vi "ROI entry-Offset ROI (core).vi"(9 "Function":T1=enum."Offset all ROI", 10 "ROI setup in":T2[](array[typedef]) {"ROI group ID" format="%#_6f"; "Laser Power (%)" format="%#_6f"; "Zoom" format="%#_6f"; "Frame Size" format="%#_6f"; "Number of lines" format="%#_6f"; "Composite ID" format="%#_6f"; "Angle (deg)" format="%#_6f"; "ROI Time (ns)" format="%#_6f"; "ROI ID" format="%#_6f"; "Pixels in ROI" format="%#_6f"; "ROI index" format="%#_6f"; "Z stop" format="%#_6f"; "Y stop" format="%#_6f"; "X stop" format="%#_6f"; "Z start" format="%#_6f"; "X start" format="%#_6f"; "Y start" format="%#_6f"}, 11 "Offsets cluster in":cluster{"X offset":dbl, "Y offset":dbl}) -> (2 "ROI setup":T2[](array[typedef]) {"ROI group ID" format="%#_6f"; "Laser Power (%)" format="%#_6f"; "Zoom" format="%#_6f"; "Frame Size" format="%#_6f"; "Number of lines" format="%#_6f"; "Composite ID" format="%#_6f"; "Angle (deg)" format="%#_6f"; "ROI Time (ns)" format="%#_6f"; "ROI ID" format="%#_6f"; "Pixels in ROI" format="%#_6f"; "ROI index" format="%#_6f"; "Z stop" format="%#_6f"; "Y stop" format="%#_6f"; "X stop" format="%#_6f"; "Z start" format="%#_6f"; "X start" format="%#_6f"; "Y start" format="%#_6f"})   [LabVIEW 2013]
uses:
  Visualisation/Functional Imaging Viewer/Typedefs/ROI parameters data type.ctl
  Typedefs/ROI management FG states.ctl
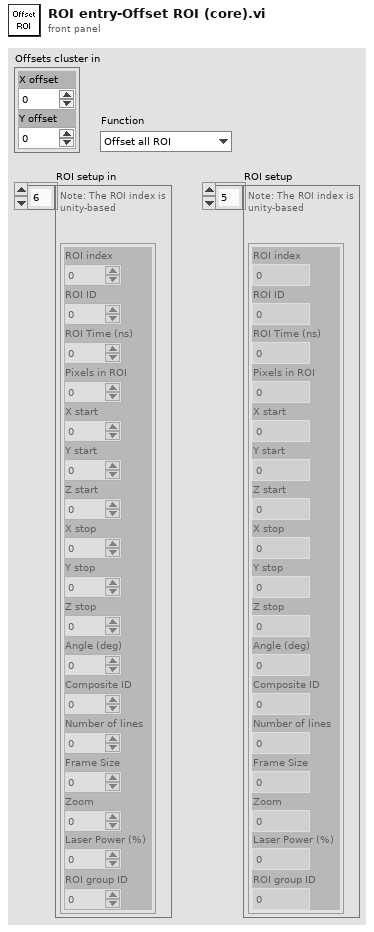
[diagram p1: front panel]
types:
  T1 = typedef "ROI management FG states.ctl" = enum16{"Read", "Write", "Clear Last", "Clear All", "Update ROIs time", "Reload last ROI set", "Offset all ROI", "Offset visible ROI"}
  T2 = typedef "ROI parameters data type.ctl" = cluster{"ROI index":dbl, "ROI ID":dbl, "ROI Time (ns)":dbl, "Pixels in ROI":dbl, "X start":dbl, "Y start":dbl, "Z start":dbl, "X stop":dbl, "Y stop":dbl, "Z stop":dbl, "Angle (deg)":dbl, "Composite ID":dbl, "Number of lines":dbl, "Frame Size":dbl, "Zoom":dbl, "Laser Power (%)":dbl, "ROI group ID":dbl}
  T3 = typedef "Offset adjustments cluster.ctl" = cluster{"X min offset":dbl, "Apply Xmin offset":bool, "X max offset":dbl, "Apply Xmax offset":bool, "Y min offset":dbl, "Apply Ymin offset":bool, "Y max offset":dbl, "Apply Ymax offset":bool}
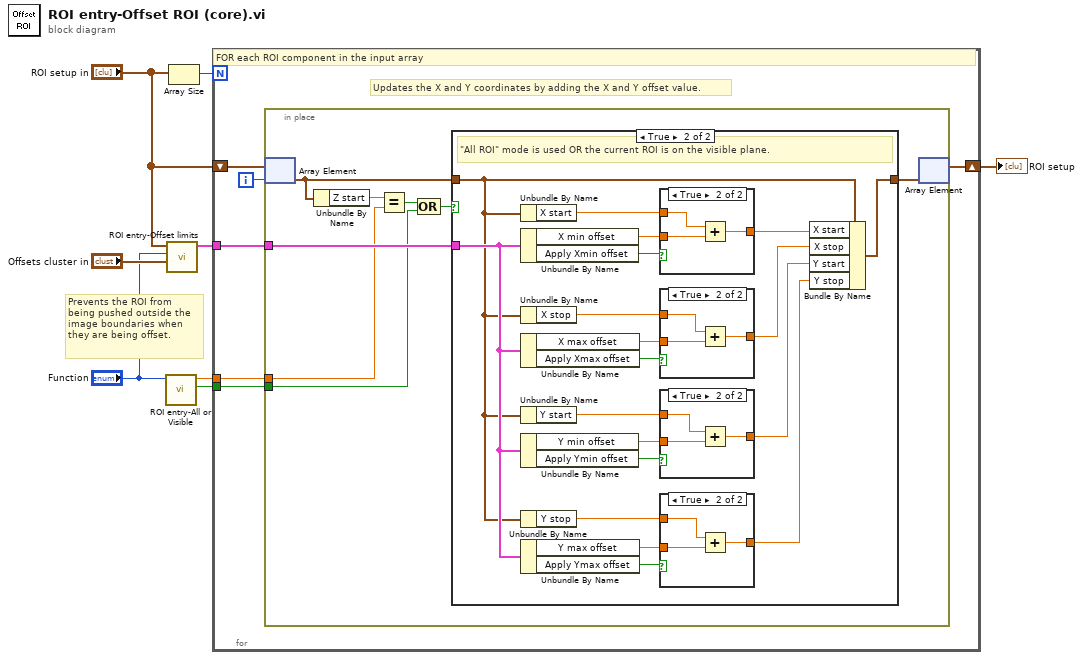
[diagram p0: block diagram]
diagram:
  # "Prevents the ROI from being pushed outside the image boundaries when they are being offset."
  n1 = call "ROI entry-All or Visible.vi"("Function"="Function") -> ("Offset ALL"=w1:bool, "Motor Z"=w2:dbl)  [unwired: 9 in]
  n2 = call "ROI entry-Offset limits.vi"("Offsets cluster in in"="Offsets cluster in", "Function"="Function", "ROI setup in"="ROI setup in") -> ("Offsets cluster out"=w7:T3)  [unwired: 8 in]
  n3 = Array Size(array="ROI setup in") -> (size(s)=w6:i32)
  n4 = for {
    N: w6 -> [_]
    shift-right: [w11] -> w8
    shift-left: "ROI setup in" -> [w14]
    tunnel: w7 -> [w12]
    tunnel: w2 -> [w10]
    tunnel: w1 -> [w9]
    i -> [w13]
    # "Updates the X and Y coordinates by adding the X and Y offset value."
    # "FOR each ROI component in the input array"
    n5 = in-place {
      in-place-border: w12 -> [w21]
      in-place-border: w10 -> [w17]
      in-place-border: w9 -> [w16]
      n6 = in-place-array #1(w14, w13) -> (w18:T2)
      n7 = Unbundle By Name(w18) -> ("Z start"=w19:dbl)
      n8 = Equal?(x=w19, y=w17) -> (x = y?=w20:bool)
      n9 = Compound Arithmetic op=OR(w20, w16) -> (w15:bool)
      n10 = case shown="True" w15 {
        tunnel: [w23 w42] -> w22
        tunnel: w21 -> [_ w41]
        tunnel: w18 -> [w23 w40]
        frame False {
        }
        frame True {
          # "\"All ROI\" mode is used OR the current ROI is on the visible plane."
          n11 = Unbundle By Name(w40) -> ("X start"=w39:dbl)
          n12 = Unbundle By Name(w41) -> ("X min offset"=w38:dbl, "Apply Xmin offset"=w36:bool)
          n13 = Unbundle By Name(w40) -> ("X stop"=w33:dbl)
          n14 = Unbundle By Name(w41) -> ("X max offset"=w34:dbl, "Apply Xmax offset"=w35:bool)
          n15 = Unbundle By Name(w40) -> ("Y start"=w32:dbl)
          n16 = Unbundle By Name(w41) -> ("Y min offset"=w31:dbl, "Apply Ymin offset"=w30:bool)
          n17 = Unbundle By Name(w40) -> ("Y stop"=w27:dbl)
          n18 = Unbundle By Name(w41) -> ("Y max offset"=w28:dbl, "Apply Ymax offset"=w29:bool)
          n19 = case shown="True" w36 {
            tunnel: w39 -> [w55 w56]
            tunnel: w38 -> [_ w57]
            tunnel: [w55 w58] -> w37
            frame False {
            }
            frame True {
              n20 = Add(x=w56, y=w57) -> (x+y=w58:dbl)
            }
          }
          n21 = case shown="True" w35 {
            tunnel: w33 -> [w51 w53]
            tunnel: w34 -> [_ w52]
            tunnel: [w51 w54] -> w26
            frame False {
            }
            frame True {
              n22 = Add(x=w53, y=w52) -> (x+y=w54:dbl)
            }
          }
          n23 = case shown="True" w30 {
            tunnel: w32 -> [w47 w49]
            tunnel: w31 -> [_ w48]
            tunnel: [w47 w50] -> w25
            frame False {
            }
            frame True {
              n24 = Add(x=w49, y=w48) -> (x+y=w50:dbl)
            }
          }
          n25 = case shown="True" w29 {
            tunnel: w27 -> [w43 w44]
            tunnel: w28 -> [_ w45]
            tunnel: [w43 w46] -> w24
            frame False {
            }
            frame True {
              n26 = Add(x=w44, y=w45) -> (x+y=w46:dbl)
            }
          }
          n27 = Bundle By Name(cluster=w40, "X start"=w37, "X stop"=w26, "Y start"=w25, "Y stop"=w24) -> (w42:T2)
        }
      }
      n28 = in-place-array #1(w22) -> (w11:T2[])  [unwired: 1 out]
    }
  }
  "ROI setup" <- w8
